vi "SHA-1 (File).vi"(10 "filepath":path) -> (2 "SHA-1 hash":string)   [LabVIEW 2013, in "SHA-1.lvlib"]
uses:
  SHA-1.lvlib
  SHA-1.lvclass
  Data-vector.ctl
  pad.vi
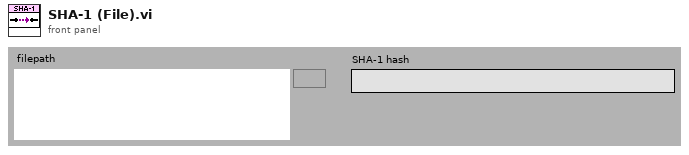
[diagram p1: front panel]
types:
  T1 = typedef "SHA-1.lvlib/SHA-1.lvclass/Data-vector.ctl" = cluster{"Data[ ]":u8[], "end":bool}
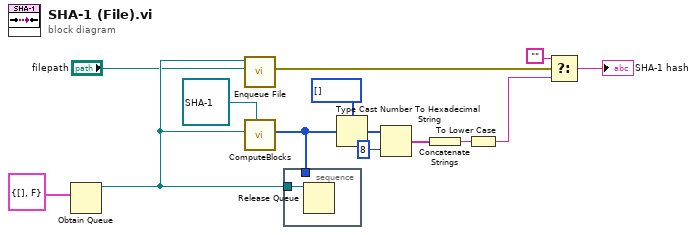
[diagram p0: block diagram]
diagram:
  n1 = Obtain Queue(element data type=T1 {"Data[ ]"=[], "end"=FALSE} ("cluster")) -> (queue out=w10:refnum<queue>)  [unwired: 4 in, 2 out]
  n2 = call "Enqueue File.vi"("filepath"="filepath", "Blocks queue"=w10) -> ("error out"=w8:errorcluster)  [unwired: 9 in]
  n3 = call-dynamic "ComputeBlocks.vi"("SHA-1"=refnum<class "SHA-1.lvclass"> refnum, "blocks queue"=w10) -> ("hash"=w1:u8[])  [unwired: 9 in]
  n4 = stacked-sequence {
    tunnel: w10 -> [w15]
    tunnel: w1 -> [_]
    frame #0 {
      n5 = Release Queue(queue=w15) -> ()  [unwired: 2 in, 3 out]
    }
  }
  n6 = Type Cast(type=u32[] [] ("U32"), x=w1) -> (*(type *) &x=w5:u32[])
  n7 = Number To Hexadecimal String(1:i16 8 ("width (-)"), 2:w5) -> (0:w4:string[])
  n8 = Concatenate Strings(w4) -> (w3:string)
  n9 = To Lower Case(string=w3) -> (all lower case string=w2:string)
  n10 = Select(t="", s=w8, f=w2) -> (s? t:f=→"SHA-1 hash":string)
